vi "Cam save image.vi"(8 "error in (no error)":errorcluster, 9 "file index":i32, 10 "page":u16[][](array[numeric]), 11 "Camera in":refnum<class "Camera.lvclass">) -> (0 "error out":errorcluster, 3 "Camera out":refnum<class "Camera.lvclass">)   [LabVIEW 2021, in "Camera.lvlib" / "Camera.lvclass"]
uses:
  Camera.lvclass
  C:/Program Files (x86)/National Instruments/LabVIEW 2021/vi.lib/ActorFramework/Actor/Actor.lvclass
  <vilib>/ActorFramework/Actor/Actor.lvclass/Actor.ctl
  Camera.lvclass/Camera.ctl
  Main_Control/Main_Control Messages/UI cam 1 frame saved Msg/UI cam 1 frame saved Msg.lvclass/UI cam 1 frame saved Msg.ctl
  <vilib>/ActorFramework/Message Enqueuer/Message Enqueuer.lvclass/Message Enqueuer.ctl
  <vilib>/ActorFramework/Message Enqueuer/Enqueue.vi
  Main_Control/Main_Control Messages/UI cam 1 frame saved Msg/UI cam 1 frame saved Msg.lvclass
  C:/Program Files (x86)/National Instruments/LabVIEW 2021/vi.lib/ActorFramework/Message/Message.lvclass
  <vilib>/ActorFramework/Message Priority Queue/Priority Enqueue.vi
  <vilib>/ActorFramework/Actor/Actor.lvclass
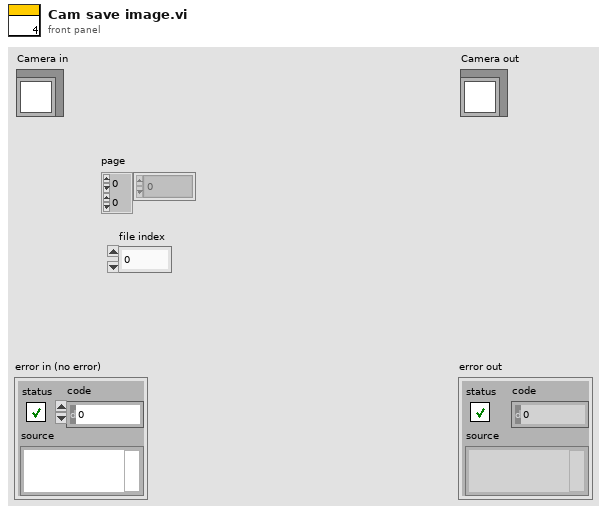
[diagram p1: front panel]
types:
  T1 = cluster{"Rows Per Strip":i32, "Photometric":i32, "Compression Type":i32}
  T2 = typedef "Image Type" = u32
  T3 = typedef "IMAQ Image.ctl" = refnum<image>
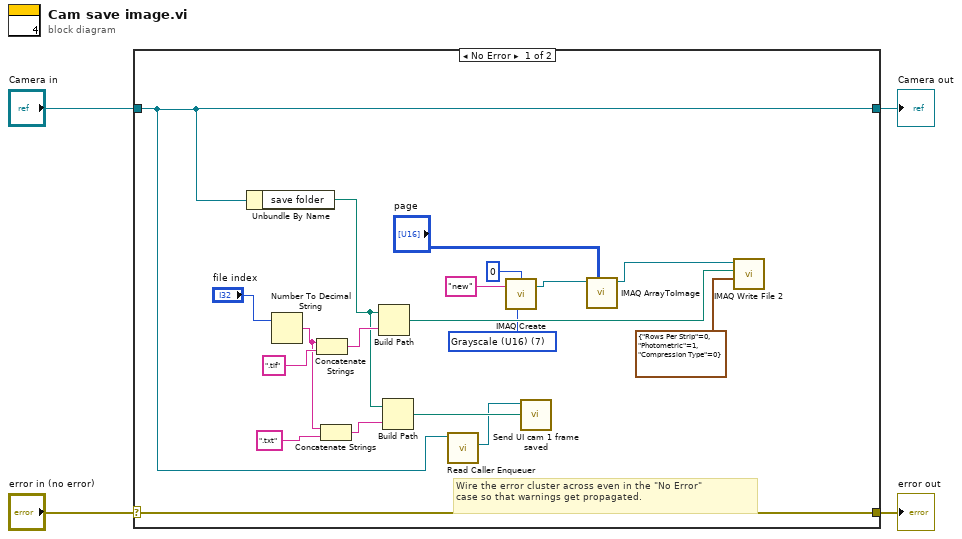
[diagram p0: block diagram]
diagram:
  n1 = case shown="No Error" "error in (no error)" {
    selector: "error in (no error)" -> [w23 w25]
    tunnel: [w23 w25] -> w3
    tunnel: [w11 w24] -> w1
    tunnel: "Camera in" -> [w11 w24]
    frame No Error {
      w8 = T2 7 items=["Grayscale (U8)", "Grayscale (I16)", "Grayscale (SGL)", "Complex (CSG)", "RGB (U32)", "HSL (U32)", "RGB (U64)", "Grayscale (U16)"] ("Image Type")
      # "Wire the error cluster across even in the \"No Error\"\ncase so that warnings get propagated."
      n2 = Unbundle By Name(w11) -> ("save folder"=w17:path)
      n3 = Number To Decimal String(number="file index") -> (decimal integer string=w15:string)  [unwired: 1 in]
      n4 = Concatenate Strings(w15, ".tif" ("string")) -> (w18:string)
      n5 = Concatenate Strings(w15, ".txt" ("string")) -> (w16:string)
      n6 = Build Path(base path=w17, name or relative path=w18) -> (appended path=w22:path)
      n7 = Build Path(base path=w17, name or relative path=w16) -> (appended path=w13:path)
      n8 = call <vilib>:"Read Caller Enqueuer.vi"("Actor"=w11) -> ("Caller Enqueuer"=w12:refnum<class "Message Enqueuer.lvclass">)  [unwired: 10 in]
      n9 = call "IMAQ Create"("Border Size"=0, "Image Name"="new", "Image Type"=w8) -> ("New Image"=w7:T3)  [unwired: 2 in, 1 out]
      n10 = call "Send UI cam 1 frame saved.vi"("file path"=w13, "Message Enqueuer"=w12) -> ()  [unwired: 8 in, 2 out]
      n11 = call "IMAQ ArrayToImage"("Image Pixels (U16)"="page", "Image"=w7) -> ("Image Out"=w5:T3)  [unwired: 8 in, 1 out]
      n12 = call-poly "IMAQ Write File 2"("TIFF Options"=T1 {"Rows Per Strip"=0, "Photometric"=1, "Compression Type"=0}, "File Path"=w22, "Image"=w5) -> ()  [unwired: 7 in, 2 out]
    }
    frame Error {
    }
  }
  "error out" <- w3
  "Camera out" <- w1
